vi "CF.vi"(5 "Display Resolution (6)":dbl=6.0, 6 "Auto Resolution (1: ON)":i32(ring)=1 items=["OFF", "ON", "ONCE"], 7 "Auto Range Value (2.0000000E+2)":dbl=200.0 format="%.7e", 8 "error in (no error)":errorcluster, 9 "Auto Range (1: ON)":i32(ring)=1 items=["OFF", "ON", "ONCE"], 10 "Measurement Function (0: Voltage)":i32(ring) items=["Voltage", "Current", "Resistance", "Charge"], 11 "VISA resource name":refnum<visa-resource-name>) -> (0 "error out":errorcluster, 3 "VISA resource name out":refnum<visa-resource-name>)   [LabVIEW 2017]
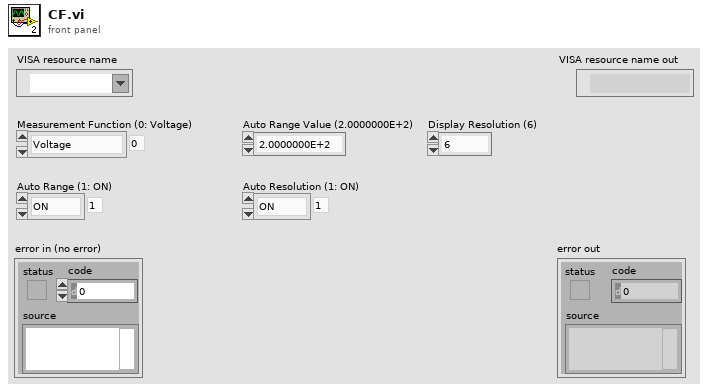
[diagram p1: front panel]
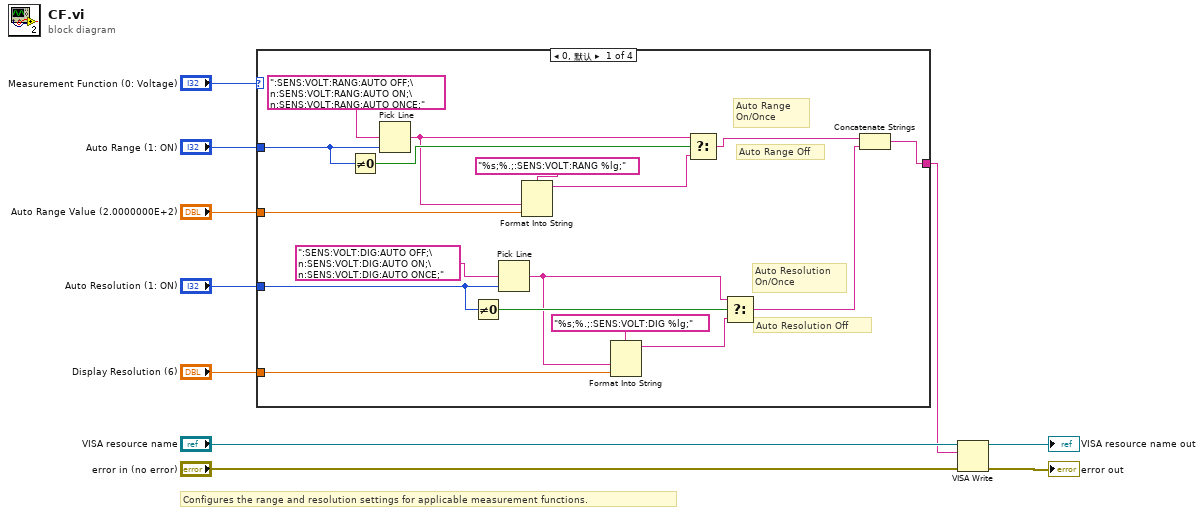
[diagram p0: block diagram]
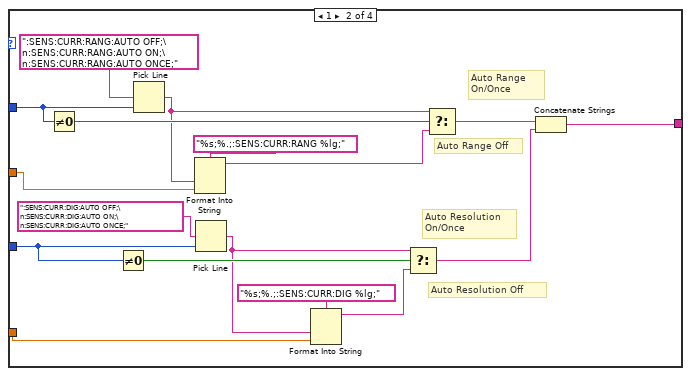
[diagram p2: hidden frame]
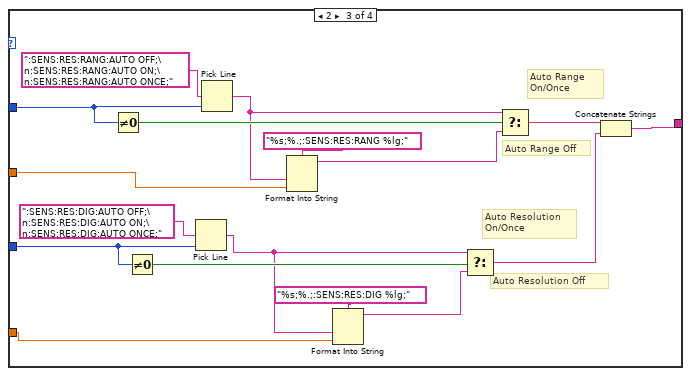
[diagram p3: hidden frame]
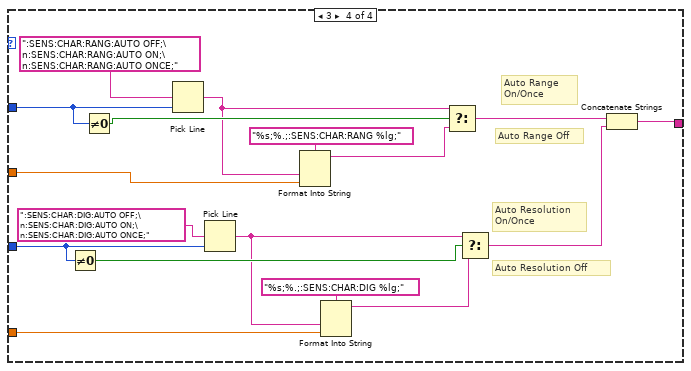
[diagram p4: hidden frame]
diagram:
  # "Configures the range and resolution settings for applicable measurement functions."
  n1 = case shown="0, 默认" "Measurement Function (0: Voltage)" {
    tunnel: "Auto Range (1: ON)" -> [w21 w43 w57 w70]
    tunnel: "Auto Range Value (2.0000000E+2)" -> [w19 w36 w50 w68]
    tunnel: "Auto Resolution (1: ON)" -> [w16 w42 w54 w65]
    tunnel: "Display Resolution (6)" -> [w13 w30 w47 w74]
    tunnel: [w22 w32 w51 w71] -> w3
    frame 0, Default {
      # "Auto Resolution Off"
      # "Auto Range Off"
      # "Auto Resolution\nOn/Once"
      # "Auto Range \nOn/Once"
      n2 = Not Equal To 0?(x=w21) -> (x != 0?=w20:bool)
      n3 = Pick Line(multi-line string=":SENS:VOLT:RANG:AUTO OFF;\n:SENS:VOLT:RANG:AUTO ON;\n:SENS:VOLT:RANG:AUTO ONCE;", line index=w21) -> (output string=w18:string)  [unwired: 1 in]
      n4 = Not Equal To 0?(x=w16) -> (x != 0?=w14:bool)
      n5 = Pick Line(multi-line string=":SENS:VOLT:DIG:AUTO OFF;\n:SENS:VOLT:DIG:AUTO ON;\n:SENS:VOLT:DIG:AUTO ONCE;", line index=w16) -> (output string=w12:string)  [unwired: 1 in]
      n6 = Format Into String(format string="%s;%.;:SENS:VOLT:RANG %lg;", w18, w19) -> (resulting string=w17:string)  [unwired: 2 in, 1 out]
      n7 = Format Into String(format string="%s;%.;:SENS:VOLT:DIG %lg;", w12, w13) -> (resulting string=w11:string)  [unwired: 2 in, 1 out]
      n8 = Select(t=w18, s=w20, f=w17) -> (s? t:f=w23:string)
      n9 = Select(t=w12, s=w14, f=w11) -> (s? t:f=w15:string)
      n10 = Concatenate Strings(w23, w15) -> (w22:string)
    }
    frame 1 {
      # "Auto Resolution Off"
      # "Auto Resolution\nOn/Once"
      # "Auto Range Off"
      # "Auto Range \nOn/Once"
      n11 = Not Equal To 0?(x=w43) -> (x != 0?=w41:bool)
      n12 = Not Equal To 0?(x=w42) -> (x != 0?=w38:bool)
      n13 = Pick Line(multi-line string=":SENS:CURR:RANG:AUTO OFF;\n:SENS:CURR:RANG:AUTO ON;\n:SENS:CURR:RANG:AUTO ONCE;", line index=w43) -> (output string=w35:string)  [unwired: 1 in]
      n14 = Format Into String(format string="%s;%.;:SENS:CURR:RANG %lg;", w35, w36) -> (resulting string=w31:string)  [unwired: 2 in, 1 out]
      n15 = Pick Line(multi-line string=":SENS:CURR:DIG:AUTO OFF;\n:SENS:CURR:DIG:AUTO ON;\n:SENS:CURR:DIG:AUTO ONCE;", line index=w42) -> (output string=w29:string)  [unwired: 1 in]
      n16 = Format Into String(format string="%s;%.;:SENS:CURR:DIG %lg;", w29, w30) -> (resulting string=w28:string)  [unwired: 2 in, 1 out]
      n17 = Select(t=w29, s=w38, f=w28) -> (s? t:f=w33:string)
      n18 = Select(t=w35, s=w41, f=w31) -> (s? t:f=w40:string)
      n19 = Concatenate Strings(w40, w33) -> (w32:string)
    }
    frame 2 {
      # "Auto Resolution Off"
      # "Auto Resolution\nOn/Once"
      # "Auto Range Off"
      # "Auto Range \nOn/Once"
      n20 = Not Equal To 0?(x=w57) -> (x != 0?=w56:bool)
      n21 = Not Equal To 0?(x=w54) -> (x != 0?=w53:bool)
      n22 = Pick Line(multi-line string=":SENS:RES:DIG:AUTO OFF;\n:SENS:RES:DIG:AUTO ON;\n:SENS:RES:DIG:AUTO ONCE;", line index=w54) -> (output string=w46:string)  [unwired: 1 in]
      n23 = Pick Line(multi-line string=":SENS:RES:RANG:AUTO OFF;\n:SENS:RES:RANG:AUTO ON;\n:SENS:RES:RANG:AUTO ONCE;", line index=w57) -> (output string=w49:string)  [unwired: 1 in]
      n24 = Format Into String(format string="%s;%.;:SENS:RES:RANG %lg;", w49, w50) -> (resulting string=w48:string)  [unwired: 2 in, 1 out]
      n25 = Format Into String(format string="%s;%.;:SENS:RES:DIG %lg;", w46, w47) -> (resulting string=w45:string)  [unwired: 2 in, 1 out]
      n26 = Select(t=w46, s=w53, f=w45) -> (s? t:f=w52:string)
      n27 = Select(t=w49, s=w56, f=w48) -> (s? t:f=w55:string)
      n28 = Concatenate Strings(w55, w52) -> (w51:string)
    }
    frame 3 {
      # "Auto Resolution Off"
      # "Auto Resolution\nOn/Once"
      # "Auto Range Off"
      # "Auto Range \nOn/Once"
      n29 = Not Equal To 0?(x=w65) -> (x != 0?=w64:bool)
      n30 = Not Equal To 0?(x=w70) -> (x != 0?=w69:bool)
      n31 = Pick Line(multi-line string=":SENS:CHAR:RANG:AUTO OFF;\n:SENS:CHAR:RANG:AUTO ON;\n:SENS:CHAR:RANG:AUTO ONCE;", line index=w70) -> (output string=w67:string)  [unwired: 1 in]
      n32 = Pick Line(multi-line string=":SENS:CHAR:DIG:AUTO OFF;\n:SENS:CHAR:DIG:AUTO ON;\n:SENS:CHAR:DIG:AUTO ONCE;", line index=w65) -> (output string=w63:string)  [unwired: 1 in]
      n33 = Format Into String(format string="%s;%.;:SENS:CHAR:RANG %lg;", w67, w68) -> (resulting string=w66:string)  [unwired: 2 in, 1 out]
      n34 = Format Into String(format string="%s;%.;:SENS:CHAR:DIG %lg;", w63, w74) -> (resulting string=w62:string)  [unwired: 2 in, 1 out]
      n35 = Select(t=w67, s=w69, f=w66) -> (s? t:f=w73:string)
      n36 = Select(t=w63, s=w64, f=w62) -> (s? t:f=w72:string)
      n37 = Concatenate Strings(w73, w72) -> (w71:string)
    }
  }
  n38 = VISA Write(VISA resource name="VISA resource name", write buffer=w3, error in (no error)="error in (no error)") -> (VISA resource name out=→"VISA resource name out":refnum<visa-resource-name>, error out=→"error out":errorcluster)  [unwired: 1 out]
